vi "weight_OHAUS.vi"(6 "Reset":bool, 7 "Stop read":bool, 10 "Tick":u32=100, 11 "PV weight":dbl caption="g" format="%#.0f") -> (3 "Q":T2 {"Q m" format="%#.0f"; "Q 4" format="%#.0f"; "dM 4" format="%#.0f"; "Q 3" format="%#.0f"; "dM 3" format="%#.0f"; "Q 2" format="%#.0f"; "dM 2" format="%#.0f"; "Q 1" format="%#.0f"; "dT 1" format="%#.0f"})   [LabVIEW 2019, in "Inputs.lvlib"]
uses:
  Inputs.lvlib
  Userlib.lvlib
panel:
  in  "Tab Control":T1(tab)=enum."Настройки"
  in  "Период 4, мин":i32=60
  in  "Период 3, мин":i32=10
  in  "Период 2, мин":i32=5
  in  "Tare":dbl caption="g" format="%#.0f"
  in  "<0>":bool
  in  "<вес>":bool
  in  "k":dbl=1.0 caption="g" format="%#.3f"
  in  "Вес":dbl caption="g" format="%#.0f"
  in  "Период обнуления, с":i32=300
  in  "Период 1, такт":i32=10
  # "время 10 g"
  # "(вес за период)"
  # "(расход)"
  # "Вес тары\n(полностью очистить бункер от продукта\nи запомнить PV weight или ввести вручную)."
  # "Вес тары\n(ввести фактический вес без учета тары\nили ввести k вручную)"
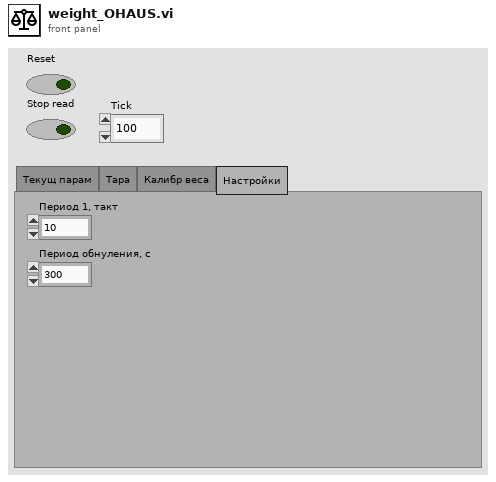
[diagram p1: front panel]
types:
  T1 = enum32{"Текущ парам", "Тара", "Калибр веса", "Настройки"}
  T2 = cluster{"Q m":dbl, "Q 1":dbl, "dT 1":dbl, "Q 2":dbl, "dM 2":dbl, "Q 3":dbl, "dM 3":dbl, "Q 4":dbl, "dM 4":dbl}
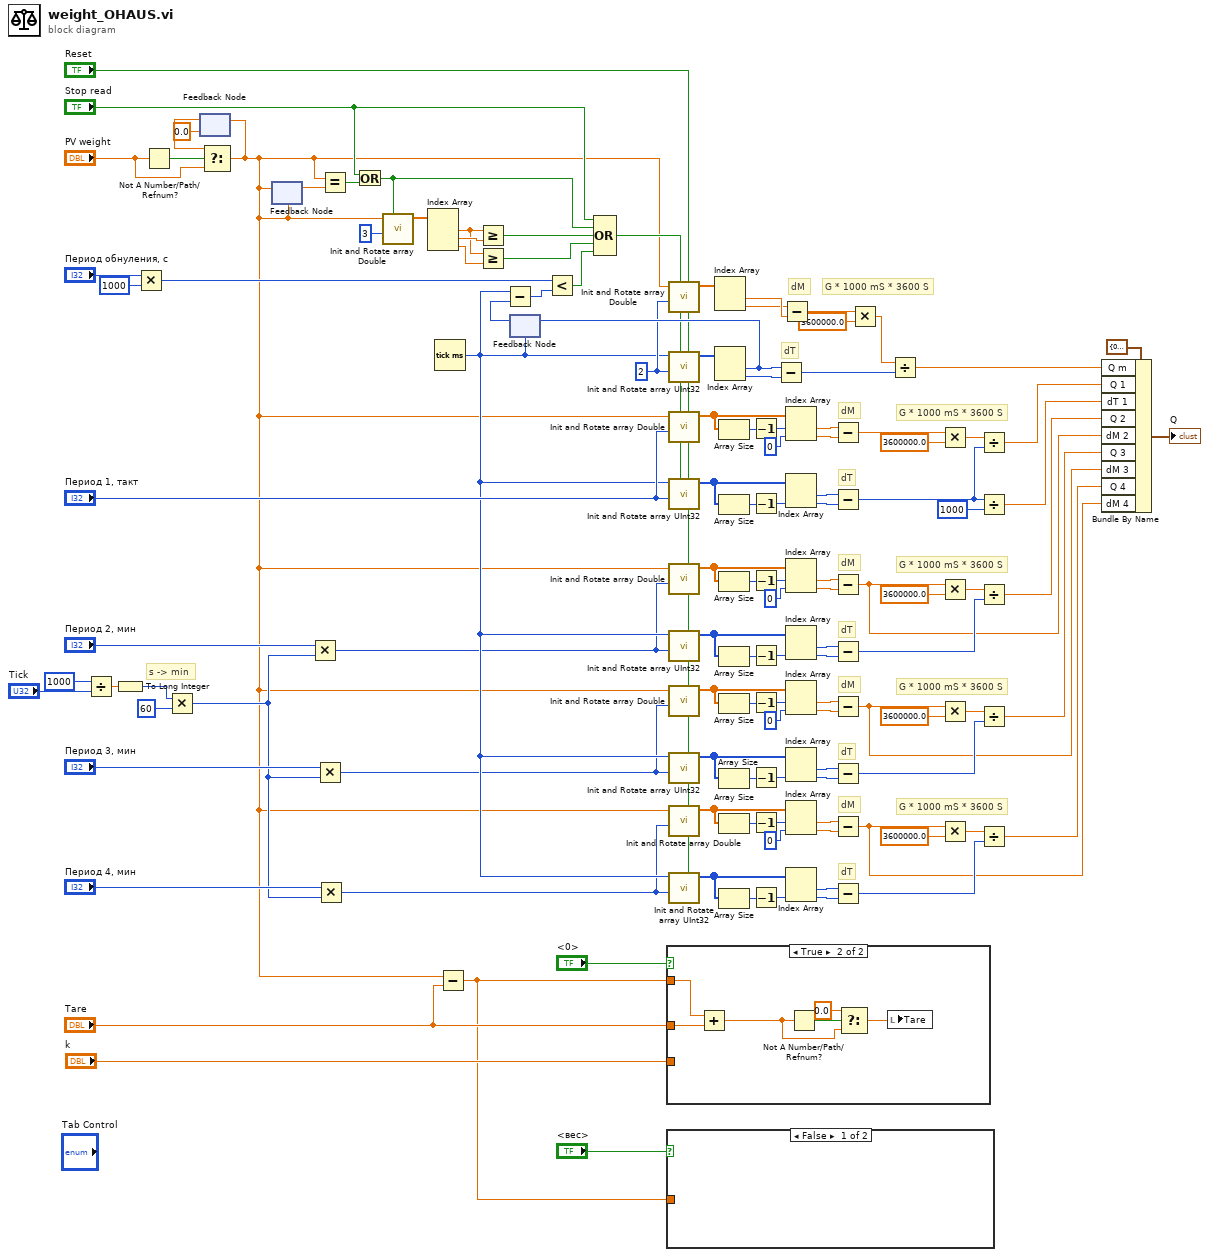
[diagram p0: block diagram]
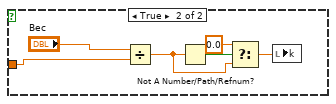
[diagram p3: hidden frame]
diagram:
  w67 = 2 ("Array size")
  # "s -> min"
  # "dT"
  # "G * 1000 mS * 3600 S"
  # "dM"
  # "dT"
  # "G * 1000 mS * 3600 S"
  # "dM"
  # "dM"
  # "G * 1000 mS * 3600 S"
  # "dT"
  # "G * 1000 mS * 3600 S"
  # "dM"
  # "dT"
  # "dT"
  # "G * 1000 mS * 3600 S"
  # "dM"
  n1 = Divide(x=1000 ("y"), y="Tick") -> (x/y=w13:dbl)
  n2 = To Long Integer(number=w13) -> (32bit integer=w9:i32)
  n3 = Multiply(x="Период обнуления, с", y=1000) -> (x*y=w93:i32)
  n4 = Not A Number/Path/Refnum?(number/path/refnum="PV weight") -> (NaN/Path/Refnum?=w5:bool)
  n5 = Multiply(x=w9, y=60) -> (x*y=w6:i32)
  n6 = feedback #1(0.0 ("f")) -> (w2:dbl)
  n7 = Select(t=w2, s=w5, f="PV weight") -> (s? t:f=w3:dbl)
  n8 = feedback-in #1(w3) -> ()
  n9 = feedback #2(w3) -> (w62:dbl)
  n10 = feedback-in #2(w3) -> ()
  n11 = Multiply(x="Период 2, мин", y=w6) -> (x*y=w11:i32)
  n12 = Multiply(x="Период 3, мин", y=w6) -> (x*y=w8:i32)
  n13 = Multiply(x="Период 4, мин", y=w6) -> (x*y=w7:i32)
  n14 = Equal?(x=w3, y=w62) -> (x = y?=w61:bool)
  n15 = Or(x="Stop read", y=w61) -> (x .or. y?=w59:bool)
  n16 = call "Init and Rotate array Double.vi"("Stop read"=w59, "Array size"=3, "PV"=w3) -> ("Array"=w102:dbl[])  [unwired: 8 in]
  n17 = Index Array(array=w102) -> (element #1=w66:dbl, element #2=w100:dbl, element #3=w65:dbl)  [unwired: 3 in]
  n18 = Tick Count (ms)() -> (millisecond timer value=w29:u32)
  n19 = Subtract(x=w3, y="Tare") -> (x-y=w119:dbl)
  n20 = Greater Or Equal?(x=w66, y=w100) -> (x >= y?=w99:bool)
  n21 = Greater Or Equal?(x=w66, y=w65) -> (x >= y?=w63:bool)
  n22 = feedback #3(w29) -> (w97:u32)
  n23 = Subtract(x=w29, y=w97) -> (x-y=w94:u32)
  n24 = Less?(x=w93, y=w94) -> (x < y?=w64:bool)
  n25 = Compound Arithmetic op=OR("Stop read", w59, w99, w63, w64) -> (w72:bool)
  n26 = case shown="True" "<0>" {
    tunnel: "Tare" -> [_ w126]
    tunnel: w119 -> [_ w125]
    tunnel: "k" -> [_ _]
    frame False {
    }
    frame True {
      n27 = Add(x=w125, y=w126) -> (x+y=w124:dbl)
      n28 = Not A Number/Path/Refnum?(number/path/refnum=w124) -> (NaN/Path/Refnum?=w129:bool)
      n29 = Select(t=0.0 ("y"), s=w129, f=w124) -> (s? t:f=w127:dbl)
      n30 = local write "Tare"(w127) -> ()
    }
  }
  n31 = case shown="False" "<вес>" {
    tunnel: w119 -> [_ w130]
    frame False {
    }
    frame True {
      n32 = Divide(x="Вес", y=w130) -> (x/y=w133:dbl)
      n33 = Not A Number/Path/Refnum?(number/path/refnum=w133) -> (NaN/Path/Refnum?=w135:bool)
      n34 = Select(t=0.0 ("y"), s=w135, f=w133) -> (s? t:f=w132:dbl)
      n35 = local write "k"(w132) -> ()
    }
  }
  n36 = call "Init and Rotate array Double.vi"("Reset"="Reset", "Stop read"=w72, "Array size"=w67, "PV"=w3) -> ("Array"=w70:dbl[])  [unwired: 7 in]
  n37 = call "Init and Rotate array UInt32.vi"("Reset"="Reset", "Stop read"=w72, "Array size"=w67, "PV"=w29) -> ("Array"=w103:u32[])  [unwired: 7 in]
  n38 = call "Init and Rotate array Double.vi"("Reset"="Reset", "Stop read"=w72, "Array size"="Период 1, такт", "PV"=w3) -> ("Array"=w116:dbl[])  [unwired: 7 in]
  n39 = call "Init and Rotate array UInt32.vi"("Reset"="Reset", "Stop read"=w72, "Array size"="Период 1, такт", "PV"=w29) -> ("Array"=w109:u32[])  [unwired: 7 in]
  n40 = call "Init and Rotate array Double.vi"("Reset"="Reset", "Array size"=w11, "PV"=w3) -> ("Array"=w81:dbl[])  [unwired: 8 in]
  n41 = call "Init and Rotate array UInt32.vi"("Reset"="Reset", "Array size"=w11, "PV"=w29) -> ("Array"=w88:u32[])  [unwired: 8 in]
  n42 = call "Init and Rotate array Double.vi"("Reset"="Reset", "Array size"=w8, "PV"=w3) -> ("Array"=w54:dbl[])  [unwired: 8 in]
  n43 = call "Init and Rotate array UInt32.vi"("Reset"="Reset", "Array size"=w8, "PV"=w29) -> ("Array"=w47:u32[])  [unwired: 8 in]
  n44 = call "Init and Rotate array Double.vi"("Reset"="Reset", "Array size"=w7, "PV"=w3) -> ("Array"=w33:dbl[])  [unwired: 8 in]
  n45 = call "Init and Rotate array UInt32.vi"("Reset"="Reset", "Array size"=w7, "PV"=w29) -> ("Array"=w40:u32[])  [unwired: 8 in]
  n46 = Index Array(array=w70) -> (element #1=w69:dbl, element #2=w68:dbl)  [unwired: 2 in]
  n47 = Index Array(array=w103) -> (element #1=w98:u32, element #2=w104:u32)  [unwired: 2 in]
  n48 = feedback-in #3(w98) -> ()
  n49 = Array Size(array=w116) -> (size(s)=w115:i32)
  n50 = Array Size(array=w109) -> (size(s)=w110:i32)
  n51 = Array Size(array=w81) -> (size(s)=w82:i32)
  n52 = Array Size(array=w88) -> (size(s)=w87:i32)
  n53 = Array Size(array=w54) -> (size(s)=w53:i32)
  n54 = Array Size(array=w47) -> (size(s)=w48:i32)
  n55 = Array Size(array=w33) -> (size(s)=w34:i32)
  n56 = Array Size(array=w40) -> (size(s)=w39:i32)
  n57 = Decrement(x=w115) -> (x-1=w112:i32)
  n58 = Decrement(x=w110) -> (x-1=w106:i32)
  n59 = Decrement(x=w82) -> (x-1=w85:i32)
  n60 = Decrement(x=w87) -> (x-1=w91:i32)
  n61 = Decrement(x=w53) -> (x-1=w50:i32)
  n62 = Decrement(x=w48) -> (x-1=w44:i32)
  n63 = Decrement(x=w34) -> (x-1=w37:i32)
  n64 = Decrement(x=w39) -> (x-1=w43:i32)
  n65 = Subtract(x=w98, y=w104) -> (x-y=w105:u32)
  n66 = Subtract(x=w68, y=w69) -> (x-y=w73:dbl)
  n67 = Index Array(array=w116, index #1=w112, index #2=0 ("index")) -> (element #1=w114:dbl, element #2=w113:dbl)
  n68 = Index Array(array=w109, index #2=w106) -> (element #1=w108:u32, element #2=w107:u32)  [unwired: 1 in]
  n69 = Index Array(array=w81, index #1=w85, index #2=0 ("index")) -> (element #1=w83:dbl, element #2=w84:dbl)
  n70 = Index Array(array=w88, index #2=w91) -> (element #1=w89:u32, element #2=w90:u32)  [unwired: 1 in]
  n71 = Index Array(array=w54, index #1=w50, index #2=0 ("index")) -> (element #1=w52:dbl, element #2=w51:dbl)
  n72 = Index Array(array=w47, index #2=w44) -> (element #1=w46:u32, element #2=w45:u32)  [unwired: 1 in]
  n73 = Index Array(array=w33, index #1=w37, index #2=0 ("index")) -> (element #1=w35:dbl, element #2=w36:dbl)
  n74 = Index Array(array=w40, index #2=w43) -> (element #1=w41:u32, element #2=w42:u32)  [unwired: 1 in]
  n75 = Subtract(x=w114, y=w113) -> (x-y=w92:dbl)
  n76 = Subtract(x=w108, y=w107) -> (x-y=w76:u32)
  n77 = Subtract(x=w83, y=w84) -> (x-y=w20:dbl)
  n78 = Subtract(x=w89, y=w90) -> (x-y=w78:u32)
  n79 = Subtract(x=w52, y=w51) -> (x-y=w18:dbl)
  n80 = Subtract(x=w46, y=w45) -> (x-y=w57:u32)
  n81 = Subtract(x=w35, y=w36) -> (x-y=w16:dbl)
  n82 = Subtract(x=w41, y=w42) -> (x-y=w30:u32)
  n83 = Multiply(x=w73, y=3600000.0) -> (x*y=w75:dbl)
  n84 = Divide(x=w75, y=w105) -> (x/y=w24:dbl)
  n85 = Multiply(x=w92, y=3600000.0) -> (x*y=w117:dbl)
  n86 = Multiply(x=w20, y=3600000.0) -> (x*y=w80:dbl)
  n87 = Multiply(x=w18, y=3600000.0) -> (x*y=w55:dbl)
  n88 = Multiply(x=w16, y=3600000.0) -> (x*y=w32:dbl)
  n89 = Divide(x=w117, y=w76) -> (x/y=w23:dbl)
  n90 = Divide(x=w76, y=u32 1000) -> (x/y=w22:dbl)
  n91 = Divide(x=w80, y=w78) -> (x/y=w21:dbl)
  n92 = Divide(x=w55, y=w57) -> (x/y=w19:dbl)
  n93 = Divide(x=w32, y=w30) -> (x/y=w17:dbl)
  n94 = Bundle By Name(cluster=T2 {"Q m"=0.0, "Q 1"=0.0, "dT 1"=0.0, "Q 2"=0.0, "dM 2"=0.0, "Q 3"=0.0, "dM 3"=0.0, "Q 4"=0.0, "dM 4"=0.0} ("Q"), "Q m"=w24, "Q 1"=w23, "dT 1"=w22, "Q 2"=w21, "dM 2"=w20, "Q 3"=w19, "dM 3"=w18, "Q 4"=w17, "dM 4"=w16) -> (→"Q":T2)
